vi "LVClass_SlopesPostProcessList Write SlopesPostProccessor.vi"(8 "error in (no error)":errorcluster, 10 "SlopesPostProcessorList":T1, 11 "SlopesPostProcessorList in":refnum<class "SlopesPostProcessorList.lvclass">) -> (0 "error out":errorcluster, 3 "SlopesPostProcessorList out":refnum<class "SlopesPostProcessorList.lvclass">)   [LabVIEW 2020, in "SlopesPostProcessorList.lvclass"]
uses:
  SlopesPostProcessorList.lvclass
  ClassID.ctl
  Handle creation.ctl
  SlopesPostProcessorList.lvclass/SlopesPostProcessorList.ctl
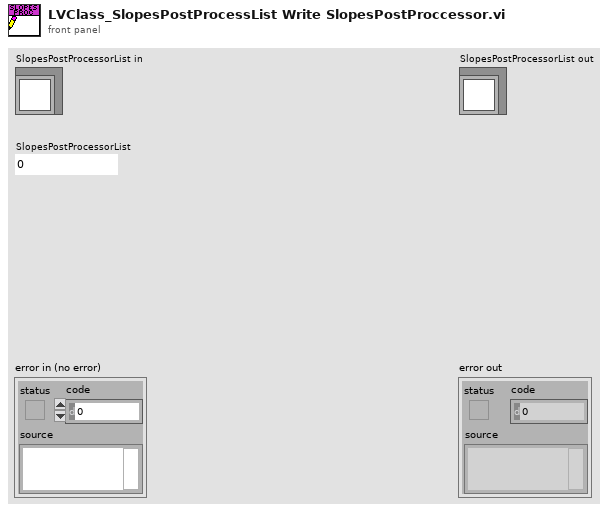
[diagram p1: front panel]
types:
  T1 = typedef "ClassID.ctl" = i64
  T2 = typedef "Handle creation.ctl" = enum16{"By ctor", "By write function"}
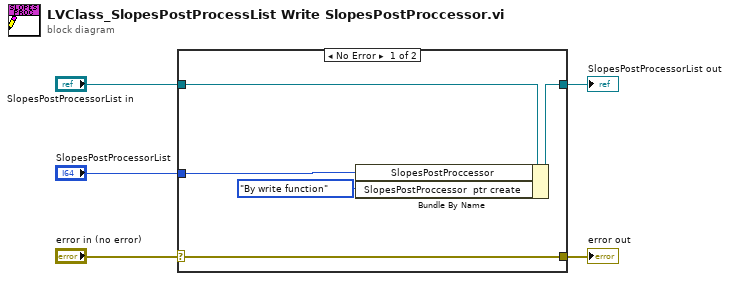
[diagram p0: block diagram]
diagram:
  n1 = case shown="No Error" "error in (no error)" {
    selector: "error in (no error)" -> [w10 w11]
    tunnel: [w10 w11] -> w4
    tunnel: [w8 w12] -> w2
    tunnel: "SlopesPostProcessorList in" -> [w9 w12]
    tunnel: "SlopesPostProcessorList" -> [w7 _]
    frame No Error {
      n2 = Bundle By Name(cluster=w9, "SlopesPostProccessor"=w7, "SlopesPostProccessor  ptr create"=Handle_creation."By write function") -> (w8:refnum<class "SlopesPostProcessorList.lvclass">)
    }
    frame Error {
    }
  }
  "error out" <- w4
  "SlopesPostProcessorList out" <- w2
